vi "UnloadExp.vi"(8 "error in (no error)":errorcluster caption="entrée d'erreur (pas d'erreur)", 11 "Experiment en entrée":refnum<class "Experiment.lvclass"> caption="DNL_LabVIEW Object in") -> (0 "error out":errorcluster caption="sortie d'erreur", 2 "SubpanelRefs":refnum<vi>[](array[refnum]), 3 "Experiment en sortie":refnum<class "Experiment.lvclass"> caption="DNL_LabVIEW Object out")   [LabVIEW 2019, in "Experiment.lvclass"]
uses:
  Experiment.lvclass
  Experiment.lvclass/Experiment.ctl
  DevicesClass/BaseDevice/BaseDevice.lvclass
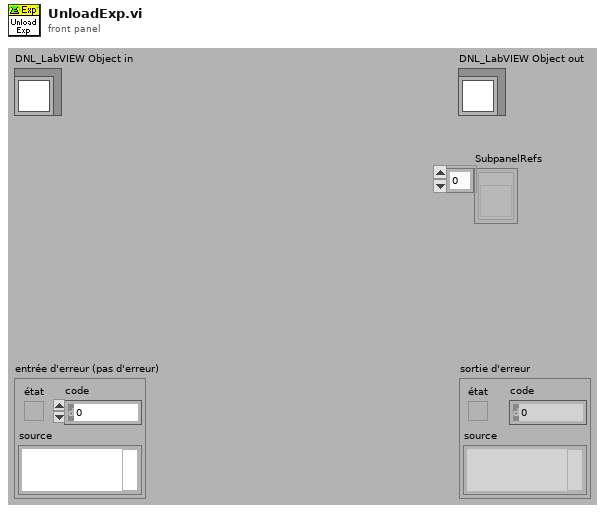
[diagram p1: front panel]
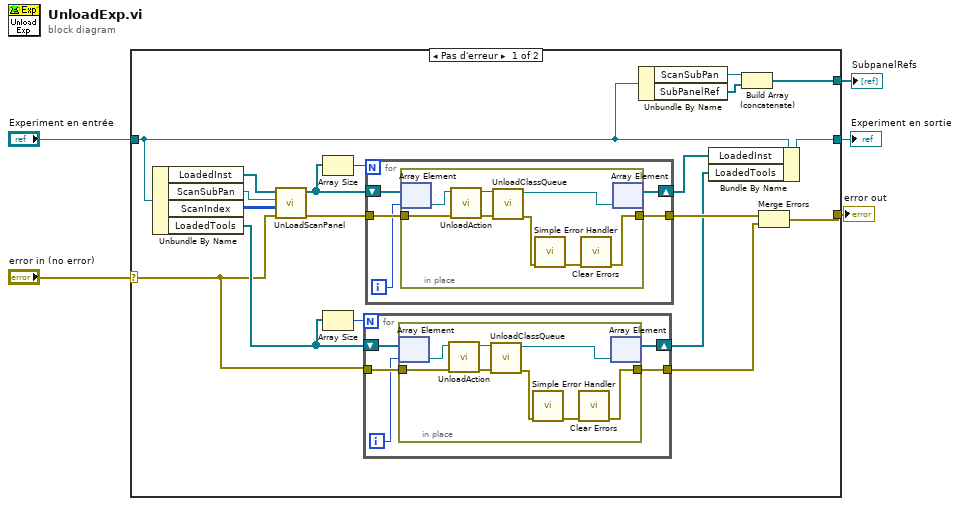
[diagram p0: block diagram]
diagram:
  n1 = case shown="Pas d'erreur" "error in (no error)" {
    selector: "error in (no error)" -> [w6 w52]
    tunnel: [w9 w52] -> w4
    tunnel: [w23 w51] -> w2
    tunnel: "Experiment en entrée" -> [w22 w51]
    tunnel: [w19 _] -> w1
    frame No Error {
      n2 = Unbundle By Name(w22) -> ("LoadedInst"=w24:refnum<class "BaseDevice.lvclass">[], "ScanSubPan"=w15:refnum<vi>, "ScanIndex"=w16:i32[][], "LoadedTools"=w12:refnum<class "BaseDevice.lvclass">[])
      n3 = call "UnLoadScanPanel.vi"("error in (no error)"=w6, "ScanIndex"=w16, "SubPanRef"=w15, "LoadedInst"=w24) -> ("sortie d'erreur"=w7:errorcluster, "LoadedInst Out"=w14:refnum<class "BaseDevice.lvclass">[])  [unwired: 6 in]
      n4 = Array Size(array=w14) -> (size(s)=w13:i32)
      n5 = Array Size(array=w12) -> (size(s)=w11:i32)
      n6 = for {
        N: w11 -> [_]
        tunnel: w6 -> [w29]
        tunnel: [w28] -> w8
        shift-right: [w25] -> w10
        shift-left: w12 -> [w27]
        i -> [w26]
        n7 = in-place {
          in-place-border: w29 -> [w37]
          in-place-border: [w32] -> w28
          n8 = in-place-array #1(w27, w26) -> (w31:refnum<class "BaseDevice.lvclass">)
          n9 = call-dynamic "UnloadAction.vi"("error in (no error)"=w37, "Device en entrée"=w31) -> ("error out"=w36:errorcluster, "Device en sortie"=w35:refnum<class "BaseDevice.lvclass">)  [unwired: 8 in]
          n10 = call "UnloadClassQueue.vi"("ErrorIn(No Error)"=w36, "BaseDevice.lvclass"=w35) -> ("sortie d'erreur"=w34:errorcluster, "BaseDevice.lvclass Out"=w30:refnum<class "BaseDevice.lvclass">)  [unwired: 8 in]
          n11 = call <vilib>:"Simple Error Handler.vi"("error in (no error)"=w34) -> ("error out"=w33:errorcluster)  [unwired: 4 in, 4 out]
          n12 = call <vilib>:"Clear Errors.vi"("error in (no error)"=w33) -> ("error out"=w32:errorcluster)  [unwired: 5 in, 1 out]
          n13 = in-place-array #1(w30) -> (w25:refnum<class "BaseDevice.lvclass">[])  [unwired: 1 out]
        }
      }
      n14 = for {
        N: w13 -> [_]
        tunnel: w7 -> [w42]
        tunnel: [w41] -> w18
        shift-right: [w38] -> w17
        shift-left: w14 -> [w40]
        i -> [w39]
        n15 = in-place {
          in-place-border: w42 -> [w50]
          in-place-border: [w45] -> w41
          n16 = in-place-array #2(w40, w39) -> (w44:refnum<class "BaseDevice.lvclass">)
          n17 = call-dynamic "UnloadAction.vi"("error in (no error)"=w50, "Device en entrée"=w44) -> ("error out"=w49:errorcluster, "Device en sortie"=w48:refnum<class "BaseDevice.lvclass">)  [unwired: 8 in]
          n18 = call "UnloadClassQueue.vi"("ErrorIn(No Error)"=w49, "BaseDevice.lvclass"=w48) -> ("sortie d'erreur"=w47:errorcluster, "BaseDevice.lvclass Out"=w43:refnum<class "BaseDevice.lvclass">)  [unwired: 8 in]
          n19 = call <vilib>:"Simple Error Handler.vi"("error in (no error)"=w47) -> ("error out"=w46:errorcluster)  [unwired: 4 in, 4 out]
          n20 = call <vilib>:"Clear Errors.vi"("error in (no error)"=w46) -> ("error out"=w45:errorcluster)  [unwired: 5 in, 1 out]
          n21 = in-place-array #2(w43) -> (w38:refnum<class "BaseDevice.lvclass">[])  [unwired: 1 out]
        }
      }
      n22 = Unbundle By Name(w22) -> ("ScanSubPan"=w21:refnum<vi>, "SubPanelRef"=w20:refnum<vi>[])
      n23 = Bundle By Name(cluster=w22, "LoadedInst"=w17, "LoadedTools"=w10) -> (w23:refnum<class "Experiment.lvclass">)
      n24 = Build Array (concatenate)(w21, w20) -> (w19:refnum<vi>[])
      n25 = Merge Errors(w18, w8) -> (w9:errorcluster)
    }
    frame Error {
    }
  }
  "error out" <- w4
  "Experiment en sortie" <- w2
  "SubpanelRefs" <- w1
